vi "Read.vi"(8 "error in (no error)":errorcluster, 9 "Timeout":i32=-1 min=-1, 10 "Number of Samples":u32=1000, 11 "AI (Continuous) Ref In":T1) -> (0 "error out":errorcluster, 2 "Values":dbl[][](array[numeric]), 3 "AI (Continuous) Ref Out":T1)   [LabVIEW 2021, in "AI Continuous.lvlib"]
doc: "Reads values from one or more analog input channels. Use this VI to read multiple samples for each channel at one time."
uses:
  <vilib>/myRIO/Instrument Drivers/Onboard IO/AI Continuous/AI Continuous.lvlib
  <vilib>/myRIO/Instrument Drivers/Onboard IO/AI Continuous/typedefs/AI Continuous Reference.ctl
  <vilib>/myRIO/Common/Instrument Driver Framework/Utilities/typedefs/myRIO Generic Hardware Reference.ctl
  <vilib>/myRIO/Common/Instrument Driver Framework/Utilities/typedefs/Hardware Version Enum.ctl
  <vilib>/myRIO/Common/Instrument Driver Framework/Utilities/typedefs/myRIO v1.0 Reference.ctl
  <vilib>/myRIO/Common/Instrument Driver Framework/Utilities/typedefs/Generic FPGA Reference.ctl
  <vilib>/myRIO/Common/Instrument Driver Framework/ELVIS III v1.0/AI Continuous/typedefs/AI Continuous Channels List.ctl
  <vilib>/myRIO/Common/Instrument Driver Framework/ELVIS III v1.0/AI Continuous/typedefs/ELVIS III v1.0 AI Continuous Channels Enum.ctl
  <vilib>/myRIO/Common/Instrument Driver Framework/Utilities/typedefs/Analog Scaling Constants.ctl
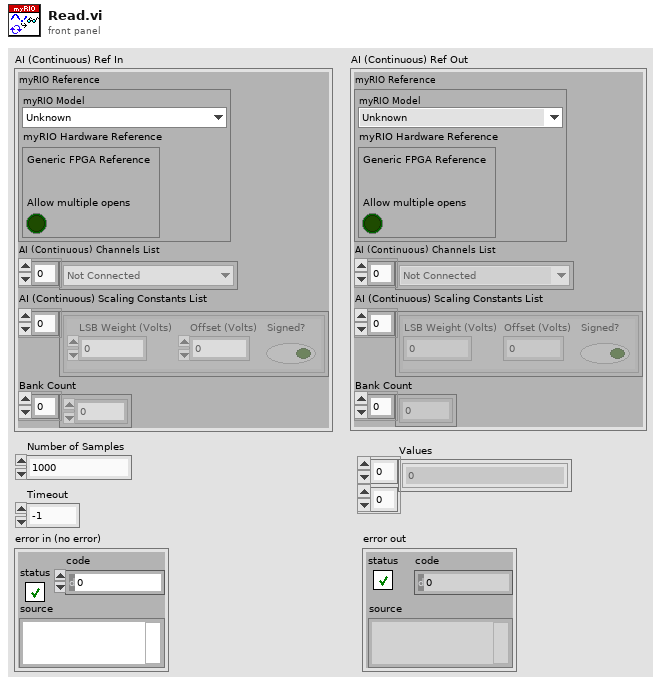
[diagram p1: front panel]
types:
  T1 = typedef "AI Continuous.lvlib/AI Continuous Reference.ctl" = cluster{"myRIO Reference":T2, "AI (Continuous) Channels List":T6, "AI (Continuous) Scaling Constants List":T8[], "Bank Count":u8[]}
  T2 = typedef "myRIO Generic Hardware Reference.ctl" = cluster{"myRIO Model":T3, "myRIO Hardware Reference":T4}
  T3 = typedef "Hardware Version Enum.ctl" = enum16{"Unknown", "myRIO-1900", "myRIO-1950", "roboRIO", "NI ELVIS RIO CM", "ELVIS III"}
  T4 = typedef "myRIO v1.0 Reference.ctl" = cluster{"Generic FPGA Reference":T5, "Allow multiple opens":bool}
  T5 = typedef "Generic FPGA Reference.ctl" = refnum<k20>
  T6 = typedef "AI Continuous Channels List.ctl" = T7[]
  T7 = typedef "ELVIS III v1.0 AI Continuous Channels Enum.ctl" = enum16{"Not Connected", "A/AI0 (Continuous)", "A/AI1 (Continuous)", "A/AI2 (Continuous)", "A/AI3 (Continuous)", "A/AI4 (Continuous)", "A/AI5 (Continuous)", "A/AI6 (Continuous)", "A/AI7 (Continuous)", "A/AI0 (DIFF Continuous)", "A/AI1 (DIFF Continuous)", "A/AI2 (DIFF Continuous)", "A/AI3 (DIFF Continuous)", "B/AI0 (Continuous)", "B/AI1 (Continuous)", "B/AI2 (Continuous)", "B/AI3 (Continuous)", "B/AI4 (Continuous)", "B/AI5 (Continuous)", "B/AI6 (Continuous)", "B/AI7 (Continuous)", "B/AI0 (DIFF Continuous)", "B/AI1 (DIFF Continuous)", "B/AI2 (DIFF Continuous)", "B/AI3 (DIFF Continuous)"}
  T8 = typedef "Analog Scaling Constants.ctl" = cluster{"LSB Weight (Volts)":dbl, "Offset (Volts)":dbl, "Signed?":bool}
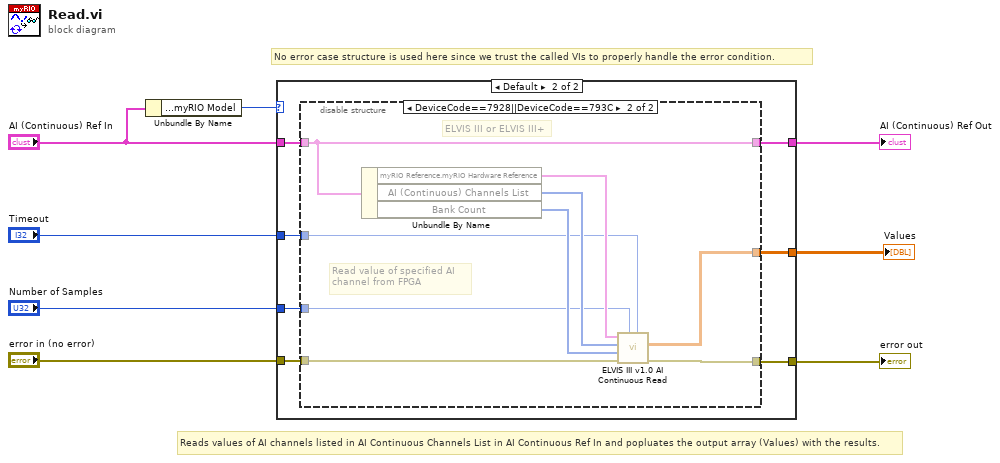
[diagram p0: block diagram]
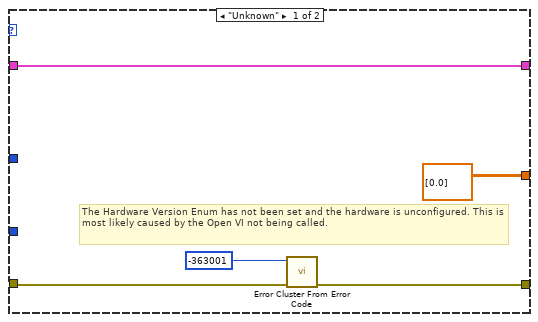
[diagram p2: hidden frame]
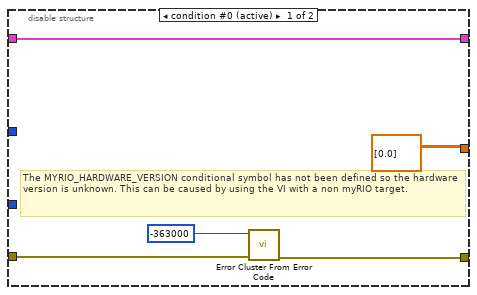
[diagram p3: hidden frame]
diagram:
  # "No error case structure is used here since we trust the called VIs to properly handle the error condition."
  # "Reads values of AI channels listed in AI Continuous Channels List in AI Continuous Ref In and popluates the output array (Values) with the results."
  n1 = Unbundle By Name("AI (Continuous) Ref In") -> ("myRIO Reference.myRIO Model"=w3:T3)
  n2 = case shown="Default" w3 {
    tunnel: [w11 w20] -> w5
    tunnel: "AI (Continuous) Ref In" -> [w10 w19]
    tunnel: "error in (no error)" -> [w12 w18]
    tunnel: [w10 w17] -> w6
    tunnel: [dbl[][] [[0.0]] w16] -> w4
    tunnel: "Number of Samples" -> [_ w15]
    tunnel: "Timeout" -> [_ w14]
    frame "Unknown" {
      # "The Hardware Version Enum has not been set and the hardware is unconfigured. This is most likely caused by the Open VI not being called."
      n3 = call <vilib>:"Error Cluster From Error Code.vi"("error in (no error)"=w12, "error code (0)"=-363001) -> ("error out"=w11:errorcluster)  [unwired: 7 in]
    }
    frame Default {
      n4 = disable-structure shown="DeviceCode==7928||DeviceCode==793C" {
        disable-tunnel: w19 -> [w22 w32]
        disable-tunnel: [w25 w30] -> w20
        disable-tunnel: w18 -> [w23 w29]
        disable-tunnel: [w22 w32] -> w17
        disable-tunnel: [dbl[][] [[0.0]] ("dbl Scaled Value List") w31] -> w16
        disable-tunnel: w15 -> [_ w27]
        disable-tunnel: w14 -> [_ w26]
        frame condition #0 (active) {
          # "The MYRIO_HARDWARE_VERSION conditional symbol has not been defined so the hardware version is unknown. This can be caused by using the VI with a non myRIO target."
          n5 = call <vilib>:"Error Cluster From Error Code.vi"("error in (no error)"=w23, "error code (0)"=-363000) -> ("error out"=w25:errorcluster)  [unwired: 7 in]
        }
        frame condition #1 {
          # "ELVIS III or ELVIS III+"
          # "Read value of specified AI \nchannel from FPGA"
          n6 = Unbundle By Name(w32) -> ("myRIO Reference.myRIO Hardware Reference"=w34:T4, "AI (Continuous) Channels List"=w33:T6, "Bank Count"=w28:u8[])
          n7 = call <vilib>:"ELVIS III v1.0 AI Continuous Read.vi"("Timeout"=w26, "Number of Samples"=w27, "error in (no error)"=w29, "Bank Count"=w28, "AI (Continuous) Channels List"=w33, "AI (Continuous) Ref In"=w34) -> ("error out"=w30:errorcluster, "Data Output"=w31:dbl[][])  [unwired: 3 in, 1 out]
        }
      }
    }
  }
  "AI (Continuous) Ref Out" <- w6
  "error out" <- w5
  "Values" <- w4
